vi "create.vi"(8 "error in (no error)":errorcluster, 10 "ref":u64) -> (0 "error out":errorcluster, 2 "item_type":T1, 3 "Item out":refnum<class "Item.lvclass">)   [LabVIEW 2020, in "toml_edit.lvlib" / "Item.lvclass"]
uses:
  Item.lvclass
  Item.lvclass/Item.ctl
  type--enum.ctl
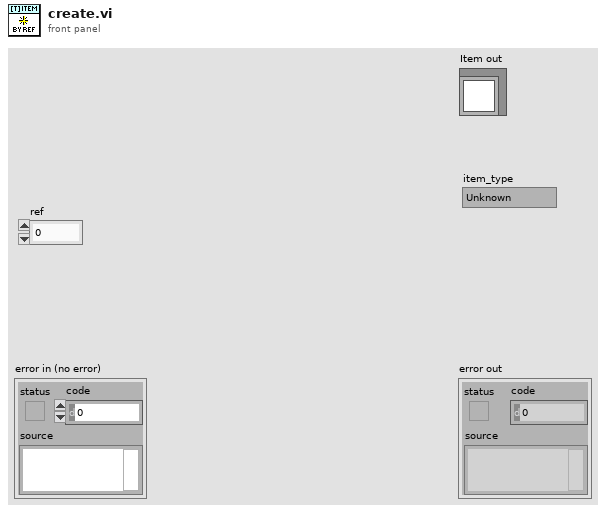
[diagram p1: front panel]
types:
  T1 = typedef "toml_edit.lvlib/Item.lvclass/type--enum.ctl" = enum16{"Unknown", "None", "Value", "ArrayOfTables", "Table"}
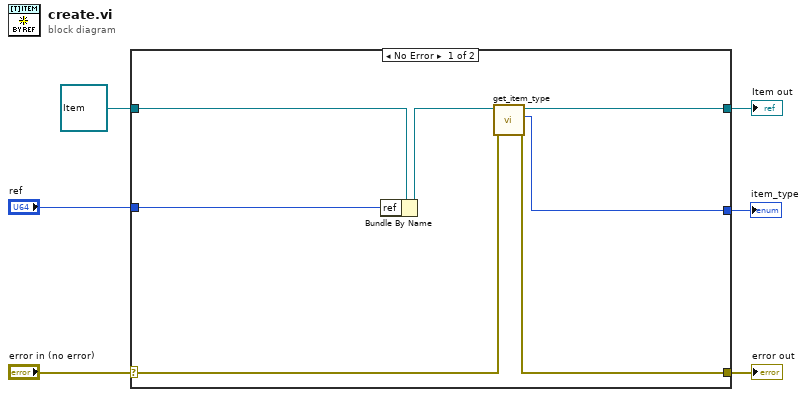
[diagram p0: block diagram]
diagram:
  n1 = case shown="No Error" "error in (no error)" {
    selector: "error in (no error)" -> [w9 w15]
    tunnel: [w8 w15] -> w5
    tunnel: [w10 w14] -> w3
    tunnel: refnum<class "Item.lvclass"> refnum ("Item in") -> [w13 w14]
    tunnel: "ref" -> [w12 _]
    tunnel: [w7 _] -> w1
    frame No Error {
      n2 = Bundle By Name(cluster=w13, "ref"=w12) -> (w11:refnum<class "Item.lvclass">)
      n3 = call "get_item_type.vi"("error in (no error)"=w9, "Item in"=w11) -> ("error out"=w8:errorcluster, "item_type"=w7:T1, "Item out"=w10:refnum<class "Item.lvclass">)  [unwired: 7 in]
    }
    frame Error {
    }
  }
  "error out" <- w5
  "Item out" <- w3
  "item_type" <- w1
